vi "TimeMeasure.vi"(8 "error in (no error)":errorcluster, 11 "time in":u32) -> (0 "error out":errorcluster, 2 "dt":u32, 3 "time out":u32)   [LabVIEW 2011]
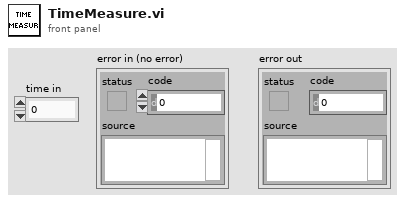
[diagram p1: front panel]
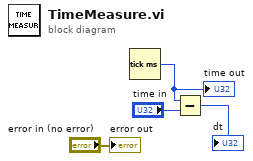
[diagram p0: block diagram]
diagram:
  n1 = Tick Count (ms)() -> (millisecond timer value=w2:u32)
  "time out" <- w2
  n2 = Subtract(x=w2, y="time in") -> (x-y=→"dt":u32)
  "error out" <- "error in (no error)"
